vi "XIPIN_AXI_Timebase_Watchdog_Timer_2_0.vi"   [LabVIEW 2017]
doc: "The Advanced eXtensible Lite (AXI) Timebase Watchdog Timer is a 32-bit peripheral that provides a 32-bit free-running timebase and watchdog timer.\n------------------------------------\n<b>Need License</b> : No\n<b>Interface</b> : AXI4"
uses:
  <vilib>/rvi/XilinxIP/XIPIN_XNode/niFpgaXIPIN.xnode
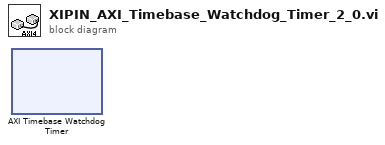
[diagram p0: block diagram]
diagram:
  n1 = xnode ("AXI Timebase Watchdog Timer")() -> ()
